vi "Pre Launch Init.vi"(11 "Generador de Señales in":refnum<class "Generador de Señales.lvclass">) -> (0 "error out":errorcluster, 3 "Generador de Señales out":refnum<class "Generador de Señales.lvclass">)   [LabVIEW 2020, in "Generador de Señales.lvlib" / "Generador de Señales.lvclass"]
doc: "(<B>Filename</B>: Actor Framework.lvlib:Actor.lvclass:Pre Launch Init.vi)\n\nDefines behavior that occurs after the Launch Nested Actor method is invoked but before the actor's Actor Core method begins running.\n\nBy default, this method does nothing. A descendant class may override it to define behavior."
uses:
  <vilib>/ActorFramework/Actor/Actor.lvclass
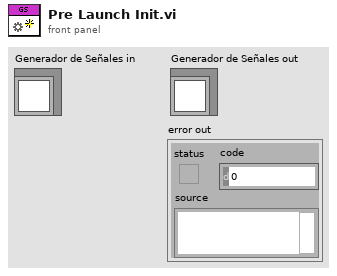
[diagram p1: front panel]
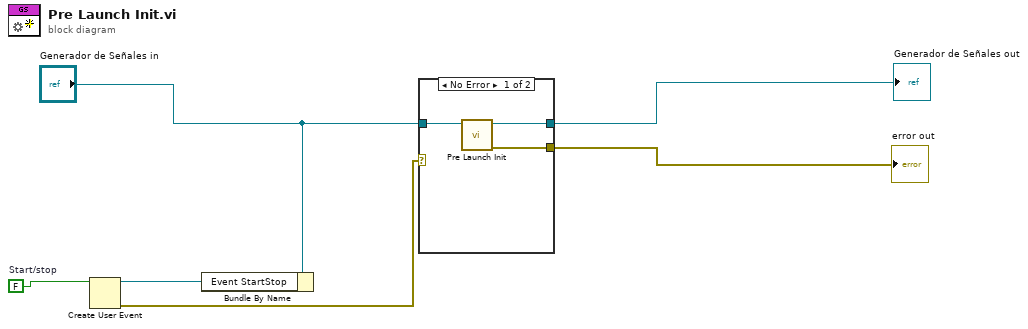
[diagram p0: block diagram]
diagram:
  w4 = FALSE  # Start/stop
  n1 = Create User Event(user event datatype=w4) -> (user event=w2:refnum<user-event>, error out=w1:errorcluster)  [unwired: 1 in]
  n2 = Bundle By Name(cluster="Generador de Señales in", "Event StartStop"=w2) -> ()  [unwired: 1 out]
  n3 = case shown="No Error" w1 {
    selector: w1 -> [_ w10]
    tunnel: [w9 w10] -> w6
    tunnel: [w8 w11] -> w5
    tunnel: "Generador de Señales in" -> [w7 w11]
    frame No Error {
      n4 = call-parent "Pre Launch Init.vi"("Actor in"=w7) -> ("error out"=w9:errorcluster, "Actor out"=w8:refnum<class "Generador de Señales.lvclass">)  [unwired: 9 in]
    }
    frame Error {
    }
  }
  "error out" <- w6
  "Generador de Señales out" <- w5
